vi "moveStageREL.vi"(1 "System no.":i32, 2 "stageIdx":i32, 3 "initPos (mm)":dbl, 4 "stage lim (mm)":dbl, 5 "Step size (mm/um)":dbl, 6 "Radio Buttons":enum32{"Coarse (mm) ", "Fine (um) "}(radio)=enum."Fine (um) ") -> (23 "stagePos":dbl)   [LabVIEW 2015]
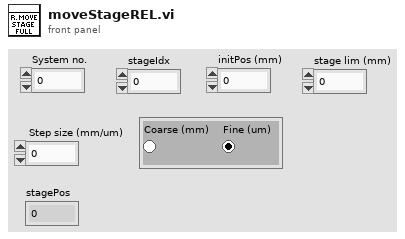
[diagram p1: front panel]
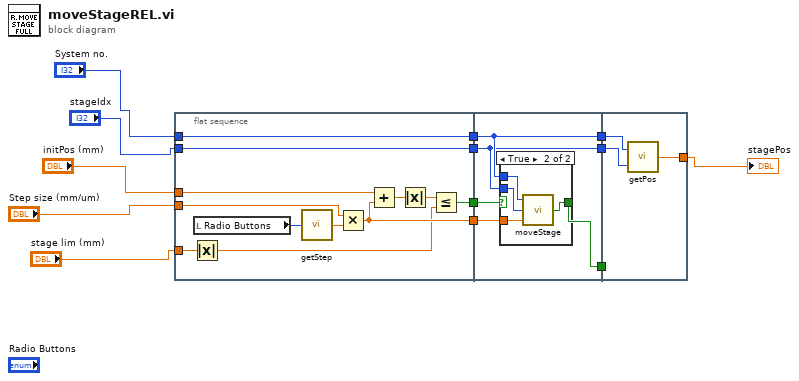
[diagram p0: block diagram]
diagram:
  n1 = flat-sequence {
    tunnel: "stageIdx" -> [w24]
    tunnel: "System no." -> [w25]
    tunnel: [w25] -> w13
    tunnel: [w24] -> w12
    tunnel: "initPos (mm)" -> [w21]
    tunnel: "stage lim (mm)" -> [w16]
    tunnel: [w20] -> w11
    tunnel: "Step size (mm/um)" -> [w19]
    tunnel: [w18] -> w10
    tunnel: [w30] -> w9
    tunnel: [w29] -> w8
    tunnel: [w28] -> w7
    tunnel: w13 -> [w29]
    tunnel: w12 -> [w28]
    tunnel: w11 -> [w27]
    tunnel: w10 -> [w26]
    tunnel: w9 -> [_]
    tunnel: w8 -> [w38]
    tunnel: w7 -> [w37]
    tunnel: [w36] -> w1
    frame #0 {
      n2 = Absolute Value(x=w16) -> (abs(x)=w14:dbl)
      n3 = local read "Radio Buttons"() -> (w22:enum32{"Coarse (mm) ", "Fine (um) "})
      n4 = call "getStep.vi"("Radio Buttons"=w22) -> ("step"=w23:dbl)
      n5 = Multiply(x=w19, y=w23) -> (x*y=w18:dbl)
      n6 = Add(x=w21, y=w18) -> (x+y=w17:dbl)
      n7 = Absolute Value(x=w17) -> (abs(x)=w15:dbl)
      n8 = Less Or Equal?(x=w15, y=w14) -> (x <= y?=w20:bool)
    }
    frame #1 {
      n9 = case shown="True" w27 {
        selector: w27 -> [w31 _]
        tunnel: [w31 w35] -> w30
        tunnel: w29 -> [_ w34]
        tunnel: w28 -> [_ w33]
        tunnel: w26 -> [_ w32]
        frame False {
        }
        frame True {
          n10 = call "moveStage.vi"("inc (mm)"=w32, "axisIdx"=w33, "System no."=w34) -> ("Stopped"=w35:bool)
        }
      }
    }
    frame #2 {
      n11 = call "getPos.vi"("axisIdx"=w37, "System no."=w38) -> ("stagePos"=w36:dbl)
    }
  }
  "stagePos" <- w1
